vi "Temperature ControlSystem with R display.vi"() -> ()   [LabVIEW 2012]
doc: "Application example"
panel:
  in  "HEATER RESISTANCE (OHMS)":dbl min=0.0 max=1000.0 step=1.0 format="%#_3f"
  in  "dR/dT":bool
  in  "SET POINT":dbl min=0.0 max=2000000.0 format="%^_5e"
  out "HEATER POWER (W)":dbl format="%^_2e"
  out "HEATER CURRENT (A)":dbl format="%^_2e"
  out "HEATER VOLTAGE (V)":dbl format="%^_2e"
  out "% OF AVAILABLE\n       POWER":dbl(knob) scale=0.0..100.0 scale format="%1d"
  out "CONTROL \n   ERROR":dbl(knob) scale=-1.0..1.0 scale format="%.1f"
  out "UPDATING\n POWER\nDISPLAYS":bool
  in  "NEXT":dbl format="%#_11g"
  in  "INTERVAL (SEC)":T1(ring)
  out "RUNNING":bool
  in  "POWER RANGE":u8(ring) items=["OFF", "1uW", "10uW", "100uW", "1mW", "10mW", "100mW", "1W", ""]
  in  "POWER BIAS":u8(ring) items=["0", "20%", "40%", "60%", "80%", "100%", ""]
  in  "DERIVATOR":u8(ring) items=["0", "1s", "2s", "5s", "10s", "20s", "50s", "100s", ""]
  in  "INTEGRATOR":u8(ring) items=["PD", "2s", "5s", "10s", "20s", "50s", "100s", "200s", "500s", "1000", "LATCHED", "PD", "N/A", "N/A", "N/A", "SHORTED", ""]
  in  "PROP.  GAIN":u8(ring) items=["5dB", "10dB", "15dB", "20dB", "25dB", "30dB", "35dB", "40dB", "45dB", "50dB", "55dB", "60dB", ""]
  in  "stop":bool
  out "MEASURED":sgl format="%^_5e"
  in  "DIGITAL REFERENCE":u16 max=19999 step=1
  in  "DISPLAY":u8(ring) items=["R", "DR", "ADJ REF", "REFERENCE", "EXC VOLT", "530A HEAT V", "530A HEAT I", "530A SET PT"]
  in  "EXCITATION":u8(ring)=7 items=["NO EXCITATION", "3 uV", "10uV", "30uV", "100uV", "300uV", "1mV", "3mV"]
  in  "RANGE":u8(ring)=3 items=["NO RANGE", "2 Ohms", "20 Ohms", "200 Ohms", "2 kOhms", "20 kOhms", "200 kOhms", "2 MOhms"]
  in  "CHANNEL":u8(ring) items=["CH0", "CH1", "CH2", "CH3", "CH4", "CH5", "CH6", "CH7"]
  in  "INPUT":u8(ring)=2 items=["ZERO", "MEAS", "CAL"]
  out "ADC OVERRANGE":bool
  # "TemperatureControlSystem with R display.vi"
  # "AVS-47B"
  # "TS-530A"
  # "Ohms"
  # "Ohms"
  # "SENSOR POLARITY"
  # "(<200R)"
  # "(Set INTERVAL to its first position if no\n TS-530A is connected)"
  # "In order to run this VI example, you need an AVS-47B and a TS-530A.  Connect the two instruments using\nthe 37-way ribbon data cable and the 30cm long BNC-BNC coaxial signal cable.  A much higher 50-ohm\ncable will have excessive capacitance => unreliable operation.  Heater resistance must remain below \n200 ohms. A 100-ohm heater is recommended, although the power meter and heater power indicator \nshow correctly also with other heater resistances.  1W power can be achieved only with a 100 ohm heater.\nWith other values, either the compliance voltage or available current will limit the power. \n\nThe sensor can have either positive or negative temperature coefficient dR/dT. Polarity must be set both\nhere on the LabView front panel and on the TS-530A physical front panel. The latter tells to the controller,\nwhether its loop gain should be positive or negative. The former is required only for the CONTROL ERROR\nmeter.  Positive deflection indicates that the power is increasing. The meter has more sensitivity in the\nmiddle for better readability near to balance.\n\nInitial parameter values are read from the configuration file. Default values will be used, if the config file\nis not found.  The last used settings are stored in the configuration file when the VI exits.  The heater\ncurrent and voltage are measured at specified intervals and the power is calculated from them.  The\nmeasurements are slow and should not be too often.  Control is not, however, affected by these\nmeasuremenst, because the analog circuitry of the TS-530A works quite independently. \n\nIn order to keep this VI rather simple, it does not offer the \"hold\" position, where control is latched\ntemporarily so that other sensors can be measured."
  # "RV-Elektroniikka Oy\nPicowatt"
  # "+"
  # "-"
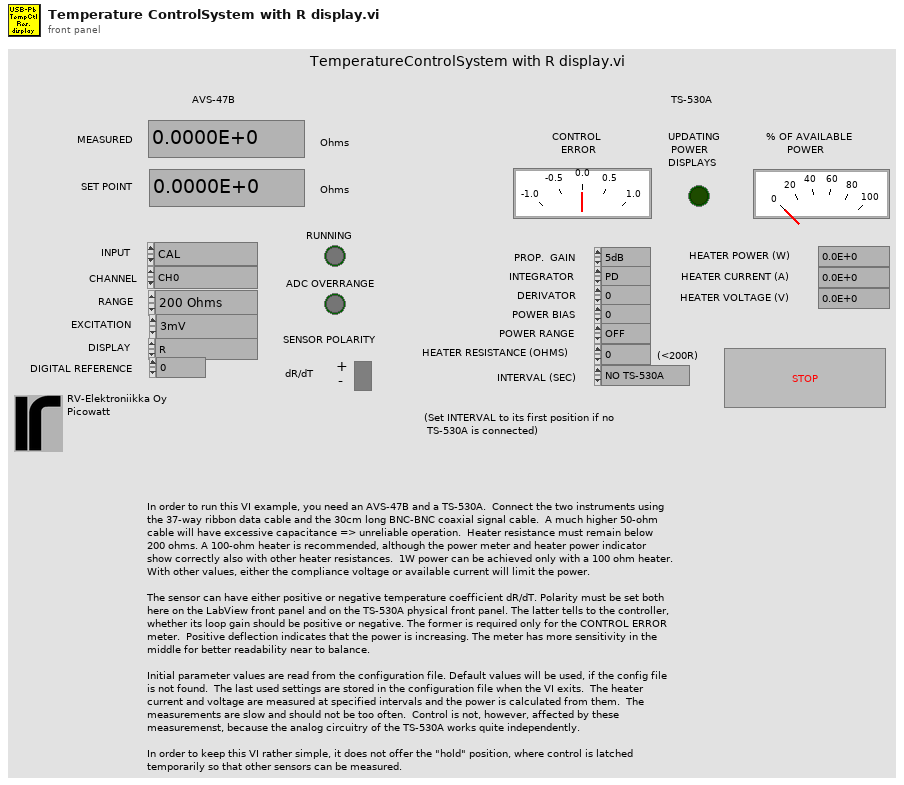
[diagram p1: front panel]
types:
  T1 = enum16{"NO TS-530A", "1", "15", "30", "45", "60"}
  T2 = cluster{"VISA RESOURCE":refnum<visa-resource-name>, "PICOBUS ADDRESS":u8, "DISABLE AL":u8, "REMOTE":u8, "INPUT":u8, "CHANNEL":u8, "RANGE":u8, "EXCITATION":u8, "DISPLAY":u8, "DIGITAL REFERENCE":u16, "SET POINT":dbl, "PROP GAIN":u8, "INTG":u8, "DERIV":u8, "POWER BIAS":u8, "POWER RANGE":u8, "INFO STRING":string, "HEATER RESISTANCE":dbl, "INTERVAL":u8, " SENSOR dR/dT":u8}
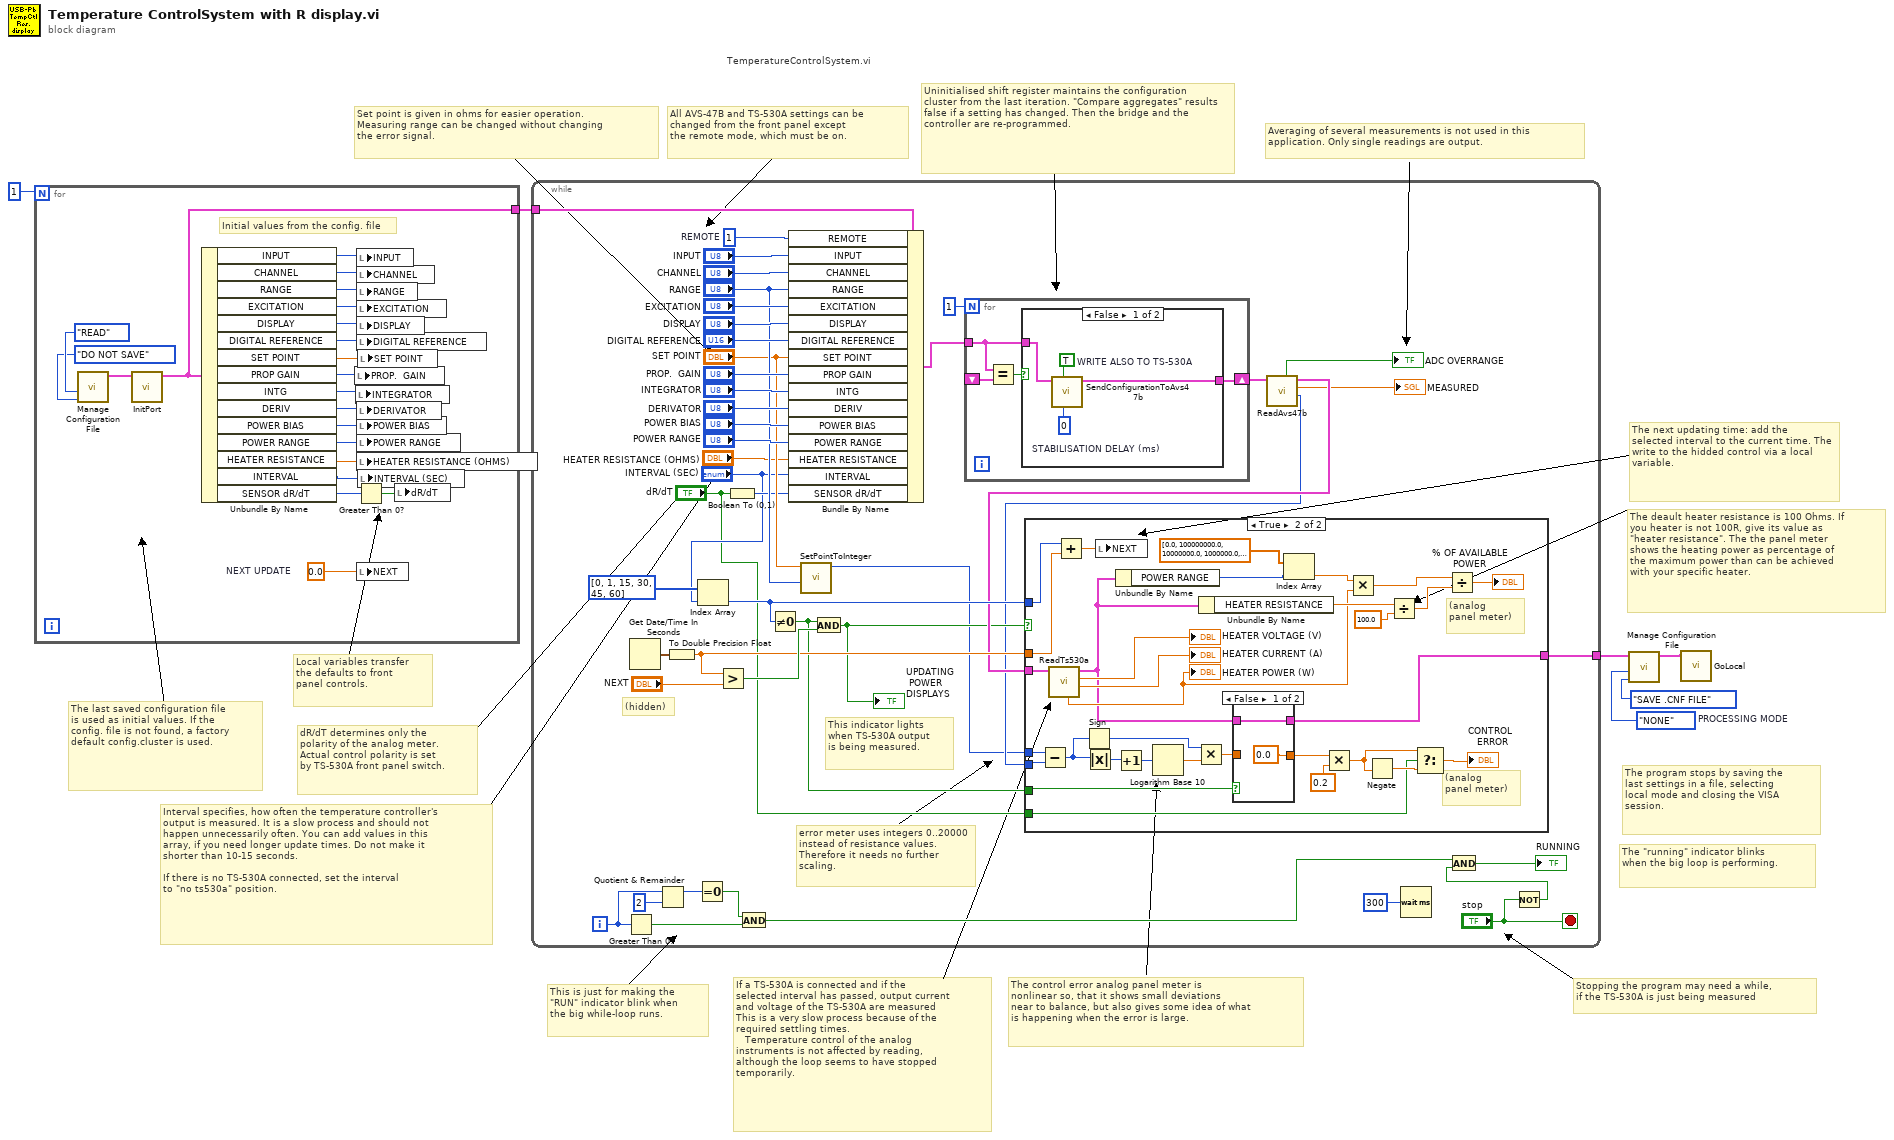
[diagram p0: block diagram]
diagram:
  w1 = enum16{"NONE", "READ", "CREATE"}."NONE"  # PROCESSING MODE
  # "TemperatureControlSystem.vi"
  # "The next updating time: add the\nselected interval to the current time. The write to the hidded control via a local variable."
  # "The program stops by saving the\nlast settings in a file, selecting\nlocal mode and closing the VISA\nsession."
  # "Stopping the program may need a while,\nif the TS-530A is just being measured"
  # "The \"running\" indicator blinks\nwhen the big loop is performing."
  # "dR/dT determines only the\npolarity of the analog meter.\nActual control polarity is set\nby TS-530A front panel switch."
  # "The deault heater resistance is 100 Ohms. If\nyou heater is not 100R, give its value as \n\"heater resistance\". The the panel meter \nshows the heating power as percentage of\nthe maximum power than can be achieved\nwith your specific heater."
  # "This is just for making the\n\"RUN\" indicator blink when\nthe big while-loop runs."
  # "The control error analog panel meter is\nnonlinear so, that it shows small deviations\nnear to balance, but also gives some idea of what\nis happening when the error is large."
  # "If a TS-530A is connected and if the\nselected interval has passed, output current\nand voltage of the TS-530A are measured\nThis is a very slow process because of the \nrequired settling times.\n   Temperature control of the analog\ninstruments is not affected by reading,\nalthough the loop seems to have stopped\ntemporarily."
  # "Interval specifies, how often the temperature controller's\noutput is measured. It is a slow process and should not \nhappen unnecessarily often. You can add values in this\narray, if you need longer update times. Do not make it\nshorter than 10-15 seconds. \n\nIf there is no TS-530A connected, set the interval\nto \"no ts530a\" position."
  # "Averaging of several measurements is not used in this\napplication. Only single readings are output."
  # "Uninitialised shift register maintains the configuration\ncluster from the last iteration. \"Compare aggregates\" results false if a setting has changed. Then the bridge and the controller are re-programmed."
  # "Set point is given in ohms for easier operation.\nMeasuring range can be changed without changing\nthe error signal."
  # "All AVS-47B and TS-530A settings can be\nchanged from the front panel except\nthe remote mode, which must be on."
  # "Local variables transfer\nthe defaults to front\npanel controls."
  # "The last saved configuration file\nis used as initial values. If the\nconfig. file is not found, a factory default config.cluster is used."
  n1 = for {
    N: 1 -> [_]
    tunnel: [w7] -> w5
    w16 = 0.0  # NEXT UPDATE
    # "Initial values from the config. file"
    n2 = call "Manage Configuration File.vi"("SAVE MODE"=enum16{"DO NOT SAVE", "SAVE .CNF FILE"}."DO NOT SAVE", "PROCESSING MODE"=enum16{"NONE", "READ", "CREATE"}."READ") -> ("CONFIGURATION CLUSTER OUT"=w8:T2)  [unwired: 9 in]
    n3 = call "InitPort.vi"("CONFIGURATION CLUSTER"=w8) -> ("UNMODIFIED CONFIGURATION CLUSTER"=w7:T2)  [unwired: 6 in, 2 out]
    n4 = Unbundle By Name(w7) -> ("INPUT"=w27:u8, "CHANNEL"=w26:u8, "RANGE"=w25:u8, "EXCITATION"=w24:u8, "DISPLAY"=w23:u8, "DIGITAL REFERENCE"=w22:u16, "SET POINT"=w11:dbl, "PROP GAIN"=w21:u8, "INTG"=w20:u8, "DERIV"=w19:u8, "POWER BIAS"=w18:u8, "POWER RANGE"=w17:u8, "HEATER RESISTANCE"=w12:dbl, "INTERVAL"=w13:u8, "SENSOR dR/dT"=w15:u8)
    n5 = local write "PROP.  GAIN"(w21) -> ()
    n6 = local write "INTEGRATOR"(w20) -> ()
    n7 = Greater Than 0?(x=w15) -> (x > 0?=w14:bool)
    n8 = local write "INPUT"(w27) -> ()
    n9 = local write "CHANNEL"(w26) -> ()
    n10 = local write "RANGE"(w25) -> ()
    n11 = local write "EXCITATION"(w24) -> ()
    n12 = local write "DISPLAY"(w23) -> ()
    n13 = local write "DIGITAL REFERENCE"(w22) -> ()
    n14 = local write "DERIVATOR"(w19) -> ()
    n15 = local write "POWER BIAS"(w18) -> ()
    n16 = local write "POWER RANGE"(w17) -> ()
    n17 = local write "HEATER RESISTANCE (OHMS)"(w12) -> ()
    n18 = local write "NEXT"(w16) -> ()
    n19 = local write "SET POINT"(w11) -> ()
    n20 = local write "INTERVAL (SEC)"(w13) -> ()
    n21 = local write "dR/dT"(w14) -> ()
  }
  n22 = while {
    tunnel: [w34] -> w3
    tunnel: w5 -> [w66]
    i -> [w54]
    stop <- "stop" stop-if-true
    w58 = u8 1  # REMOTE
    # "error meter uses integers 0..20000\ninstead of resistance values. \nTherefore it needs no further\nscaling."
    # "This indicator lights\nwhen TS-530A output\nis being measured."
    # "(hidden)"
    n23 = Greater Than 0?(x=w54) -> (x > 0?=w50:bool)
    n24 = Get Date/Time In Seconds() -> (seconds since 1Jan1904=w46:timestamp)
    n25 = Quotient & Remainder(x=w54, y=2) -> (x-y*floor(x/y)=w52:i32)  [unwired: 1 out]
    n26 = To Double Precision Float(number=w46) -> (double precision float=w43:dbl)
    n27 = Equal To 0?(x=w52) -> (x = 0?=w51:bool)
    n28 = Index Array(array=i32[] [0, 1, 15, 30, 45, 60], index="INTERVAL (SEC)") -> (element=w42:i32)
    n29 = Greater?(x=w43, y="NEXT") -> (0:w44:bool)
    n30 = Boolean To (0,1)(Boolean="dR/dT") -> (0, 1=w31:i16)
    n31 = And(x=w51, y=w50) -> (x .and. y?=w49:bool)
    n32 = Not Equal To 0?(x=w42) -> (x != 0?=w38:bool)
    n33 = Bundle By Name(cluster=w66, "REMOTE"=w58, "INPUT"="INPUT", "CHANNEL"="CHANNEL", "RANGE"="RANGE", "EXCITATION"="EXCITATION", "DISPLAY"="DISPLAY", "DIGITAL REFERENCE"="DIGITAL REFERENCE", "SET POINT"="SET POINT", "PROP GAIN"="PROP.  GAIN", "INTG"="INTEGRATOR", "DERIV"="DERIVATOR", "POWER BIAS"="POWER BIAS", "POWER RANGE"="POWER RANGE", "HEATER RESISTANCE"="HEATER RESISTANCE (OHMS)", "INTERVAL"="INTERVAL (SEC)", "SENSOR dR/dT"=w31) -> (w59:T2)
    n34 = call "SetPointToInteger.vi"("RANGE"="RANGE", "SP OHMS"="SET POINT") -> ("SP INTEGER"=w35:u16)  [unwired: 9 in]
    n35 = And(x=w38, y=w44) -> (x .and. y?=w37:bool)
    "UPDATING\n POWER\nDISPLAYS" <- w37
    n36 = for {
      N: 1 -> [_]
      shift-right: [w110] -> w48
      shift-left: _ -> [w113]
      tunnel: w59 -> [w111]
      n37 = Equal?(x=w111, y=w113) -> (x = y?=w112:bool)
      n38 = case shown="False" w112 {
        tunnel: w111 -> [w115 w118]
        tunnel: [w114 w118] -> w110
        frame False {
          w116 = TRUE  # WRITE ALSO TO TS-530A
          w117 = 0  # STABILISATION DELAY (ms)
          n39 = call "SendConfigurationToAvs47b.vi"("STABILISATION DELAY (ms)"=w117, "WRITE ALSO TO TS-530A"=w116, "CONFIGURATION CLUSTER"=w115) -> ("UNMODIFIED CONFIGURATION CLUSTER"=w114:T2)  [unwired: 5 in, 3 out]
        }
        frame True {
        }
      }
    }
    n40 = call "ReadAvs47b.vi"("CONFIGURATION CLUSTER"=w48) -> ("ADC"=w36:i32, "RESISTANCE (OHMS)"=→"MEASURED":sgl, "MODIFIED CONFIGURATION CLUSTER"=w41:T2, "ADC OVERRANGE"=→"ADC OVERRANGE":bool)  [unwired: 5 in, 2 out]
    n41 = case shown="True" w37 {
      tunnel: w42 -> [_ w105]
      tunnel: w43 -> [_ w104]
      tunnel: w41 -> [w73 w102]
      tunnel: w38 -> [_ w93]
      tunnel: w35 -> [_ w92]
      tunnel: w36 -> [_ w91]
      tunnel: "dR/dT" -> [_ w85]
      tunnel: [w73 w74] -> w34
      frame False {
      }
      frame True {
        # "(analog\npanel meter)"
        # "(analog\npanel meter)"
        n42 = Subtract(x=w92, y=w91) -> (x-y=w100:i32)
        n43 = call "ReadTs530a.vi"("CONFIGURATION CLUSTER"=w102) -> ("HEATER CURRENT"=→"HEATER CURRENT (A)":dbl, "HEATER VOLTAGE"=→"HEATER VOLTAGE (V)":dbl, "UNMODIFIED CONFIGURATION CLUSTER"=w75:T2, "HEATER POWER"=w76:dbl)  [unwired: 6 in, 1 out]
        "HEATER POWER (W)" <- w76
        n44 = Add(x=w105, y=w104) -> (x+y=w103:dbl)
        n45 = Sign(1:w100) -> (0:w99:i32)
        n46 = Absolute Value(x=w100) -> (abs(x)=w97:i32)
        n47 = local write "NEXT"(w103) -> ()
        n48 = Unbundle By Name(w75) -> ("POWER RANGE"=w83:u8)
        n49 = Increment(x=w97) -> (x+1=w96:i32)
        n50 = Logarithm Base 10(1:w96) -> (0:w98:dbl)
        n51 = Multiply(x=w99, y=w98) -> (x*y=w95:dbl)
        n52 = Unbundle By Name(w75) -> ("HEATER RESISTANCE"=w77:dbl)
        n53 = case shown="False" w93 {
          tunnel: w95 -> [_ w109]
          tunnel: [0.0 w109] -> w94
          tunnel: w75 -> [w106 w108]
          tunnel: [w106 w108] -> w74
          frame False {
          }
          frame True {
          }
        }
        n54 = Index Array(array=dbl[] [0.0, 100000000.0, 10000000.0, 1000000.0, 100000.0, 10000.0, 1000.0, 100.0], index=w83) -> (element=w82:dbl)
        n55 = Multiply(x=w94, y=0.2) -> (x*y=w87:dbl)
        n56 = Multiply(x=w82, y=w76) -> (x*y=w79:dbl)
        n57 = Negate(x=w87) -> (-x=w86:dbl)
        n58 = Divide(x=w77, y=100.0) -> (x/y=w80:dbl)
        n59 = Select(t=w87, s=w85, f=w86) -> (s? t:f=→"CONTROL \n   ERROR":dbl)
        n60 = Divide(x=w79, y=w80) -> (x/y=→"% OF AVAILABLE\n       POWER":dbl)
      }
    }
    n61 = Wait (ms)(milliseconds to wait=u32 300) -> ()  [unwired: 1 out]
    n62 = Not(x="stop") -> (.not. x?=w55:bool)
    n63 = And(x=w49, y=w55) -> (x .and. y?=→"RUNNING":bool)
  }
  n64 = call "Manage Configuration File.vi"("SAVE MODE"=enum16{"DO NOT SAVE", "SAVE .CNF FILE"}."SAVE .CNF FILE", "PROCESSING MODE"=w1, "CONFIGURATION CLUSTER"=w3) -> ("CONFIGURATION CLUSTER OUT"=w4:T2)  [unwired: 8 in]
  n65 = call "GoLocal.vi"("CONFIGURATION CLUSTER"=w4) -> ()  [unwired: 10 in, 1 out]
